vi "DFD NStage MRate Filtering with State (Wfm).vi"(6 "state in":cluster{"state ":dbl[]}[](array[cluster]), 8 "error in (no error)":errorcluster, 10 "multirate filters":T1[](array[typedef]) {"mMRate_SumWl" min=1 max=32 step=1; "mMRate_InputIwl" min=1 max=32 step=1; "mMRate_GainWl" min=1 max=32 step=1; "mMRate_OutputWl" min=1 max=32 step=1; "mMRate_InputWl" min=1 max=32 step=1; "mMRate_CoefWl" min=1 max=32 step=1; "mMRate_Mode" items=["Default"=-1, "No Rate Change"=0, "Interpolation"=1, "Decimation"=2, "Interpolated"=3, "Rational"=4]}, 11 "signal in":waveform(dbl)={"t0"=timestamp(0 s since 1904-01-01), "dt"=0.0, "Y"=[]}) -> (0 "error out":errorcluster, 3 "signal out":waveform(dbl), 4 "state out":cluster{"state ":dbl[]}[](array[cluster]))   [LabVIEW 2017, in "NI_DigFilterLicensed.lvlib"]
doc: "Filters a signal with a multistage multirate filter. You must specify the initial internal states in <B>state in</B> to filter the samples accurately. Wire data to the <B>signal in</B> input to determine the polymorphic instance to use or manually select the instance."
uses:
  <vilib>/addons/Digital Filter Design/NI_DigFilterLicensed.lvlib
  <vilib>/addons/Digital Filter Design/_Objects.llb/DFD Multirate Filter Obj.ctl
  <vilib>/addons/Digital Filter Design/_Objects.llb/DFD Multirate Mode.ctl
  <vilib>/addons/Digital Filter Design/_Objects.llb/DFD Coef Norm Type.ctl
  <vilib>/addons/Digital Filter Design/_Objects.llb/DFD Round-off Mode.ctl
  <vilib>/addons/Digital Filter Design/_Objects.llb/DFD FXP MRate Multiply Mode.ctl
  <vilib>/addons/Digital Filter Design/NI_DigFilter_Process.lvlib
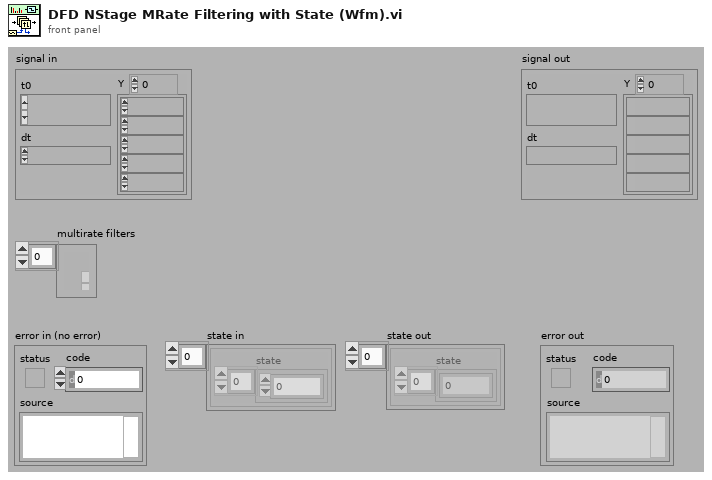
[diagram p1: front panel]
types:
  T1 = typedef "NI_DigFilterLicensed.lvlib/DFD Multirate Filter Obj.ctl" = cluster{"mMRate_Structure":enum16{"CIC", "FIR", "IIR", "Lattice"}, "mMRate_Mode":T2, "mMRate_Factor":i32, "mMRate_FIRParams":cluster{"mMRate_FIR_H":dbl[], "mMRate_FIR_IsNyquist?":bool, "mMRate_FIR_IsSymmetric?":bool}, "mMRate_CICParams":cluster{"mMRate_CIC_#Stage":i32, "mMRate_CIC_Lag":i32, "mMRate_CIC_Type":enum16{"Lowpass", "Highpass"}}, "mMRate_Order":i32, "mMRate_Version":string, "mMRate_Comments":string, "mMRate_RationalFactor":cluster{"mMRate_L":i32, "mMRate_M":i32}, "mMRate_Fs":dbl, "mMRate_Quantized?":bool, "mMRate_QFilterGain":dbl, "mMRate_CoefWl":i16, "mMRate_Scaling":cluster{"mMRate_ScaleByPowerOf2?":bool, "mMRate_ScaleType":T3}, "mMRate_InputWl":i16, "mMRate_OutputWl":i16, "mMRate_OutputMode":T4, "mMRate_MultMode":T5, "mMRate_BitPruning":bool, "mMRate_GainWl":i16, "mMRate_OutputFwl":i16, "mMRate_SumIwl":i16, "mMRate_InputIwl ":i16, "mMRate_SumWl":i16, "mMRate_CoefIwl":i16}
  T2 = typedef "NI_DigFilterLicensed.lvlib/DFD Multirate Mode.ctl" = i16
  T3 = typedef "NI_DigFilterLicensed.lvlib/DFD Coef Norm Type.ctl" = enum16{"No Norm", "Time Domain 1-Norm", "Time Domain 2-Norm", "Time Domain Inf-Norm"}
  T4 = typedef "NI_DigFilterLicensed.lvlib/DFD Round-off Mode.ctl" = enum16{"Nearest", "Truncation"}
  T5 = typedef "NI_DigFilterLicensed.lvlib/DFD FXP MRate Multiply Mode.ctl" = enum16{"Truncated", "Full"}
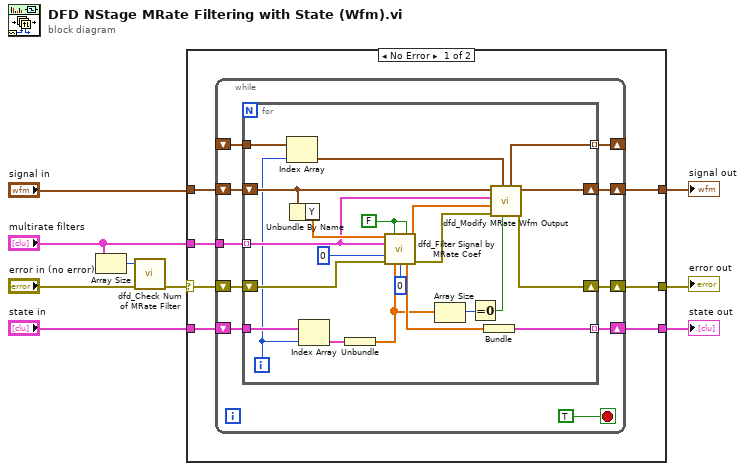
[diagram p0: block diagram]
diagram:
  n1 = Array Size(array="multirate filters") -> (size(s)=w1:i32)
  n2 = call <vilib>:"dfd_Check Num of MRate Filter.vi"("error in (no error)"="error in (no error)", "#MRate in"=w1) -> ("error out"=w2:errorcluster)  [unwired: 9 out]
  n3 = case shown="No Error" w2 {
    selector: w2 -> [w13 w49]
    tunnel: [w12 w49] -> w7
    tunnel: "multirate filters" -> [w14 _]
    tunnel: "signal in" -> [w16 _]
    tunnel: [w15 _] -> w9
    tunnel: "state in" -> [w11 _]
    tunnel: [w10 _] -> w5
    frame No Error {
      n4 = while {
        tunnel: w14 -> [w24]
        shift-right: [w17] -> _
        shift-left: _ -> [w18]
        shift-right: [w25] -> w15
        shift-left: w16 -> [w26]
        shift-right: [w22] -> w12
        shift-left: w13 -> [w23]
        shift-right: [w20] -> w10
        shift-left: w11 -> [w21]
        stop <- TRUE stop-if-true
        n5 = for {
          tunnel: w24 -> [w36] mode=indexing
          tunnel: [w47] -> w20 mode=indexing
          tunnel: w21 -> [w46]
          shift-right: [w38] -> w25
          shift-left: w26 -> [w39]
          shift-right: [w34] -> w22
          shift-left: w23 -> [w40]
          tunnel: w18 -> [w30]
          tunnel: [w28] -> w17 mode=indexing
          i -> [w27]
          w45 = FALSE ("initH?")
          n6 = Index Array(array=w30, index=w27) -> (element=w29:timestamp)
          n7 = Unbundle By Name(w39) -> ("Y"=w41:dbl[])
          n8 = Index Array(array=w46, index=w27) -> (element=w48:cluster{"state out":dbl[]})
          n9 = Unbundle(w48) -> ("state out"=w33:dbl[])
          n10 = call <vilib>:"dfd_Filter Signal by MRate Coef.vi"("signal in"=w41, "initH?"=w45, "zeroPhaseH?"=w45, "multirate filter"=w36, "skipPoint In"=0, "error in (no error)"=w40, "state in"=w33, "outputPhase"=0) -> ("signal out"=w37:dbl[], "state out"=w42:dbl[], "error out"=w35:errorcluster)  [unwired: 5 out]
          n11 = Array Size(array=w33) -> (size(s)=w32:i32)
          n12 = Equal To 0?(x=w32) -> (x = 0?=w31:bool)
          n13 = Bundle("state out"=w42) -> (w47:cluster{"state out":dbl[]})  [unwired: 1 in]
          n14 = call <vilib>:"dfd_Modify MRate Wfm Output.vi"("initH"=w31, "t0"=w29, "error in (no error)"=w35, "y"=w37, "multirate filter in"=w36, "x"=w39) -> ("error out"=w34:errorcluster, "y"=w38:waveform(dbl), "tf"=w28:timestamp)  [unwired: 3 out]
        }
      }
    }
    frame Error {
    }
  }
  "error out" <- w7
  "signal out" <- w9
  "state out" <- w5
